vi "Duplicate_AO_WF.vi"(8 "error in (no error)":errorcluster) -> (0 "error out":errorcluster)   [LabVIEW 2025]
uses:
  <vilib>/Waveform/WDTOps.llb/WDT Append Waveforms DBL.vi
panel:
  out "AO WF":waveform(dbl)[](graph) caption="Output Waveform"
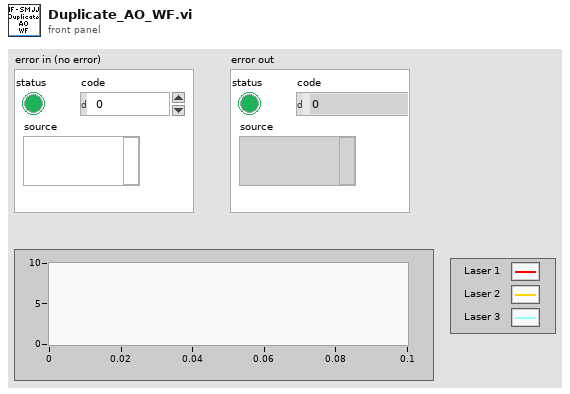
[diagram p1: front panel]
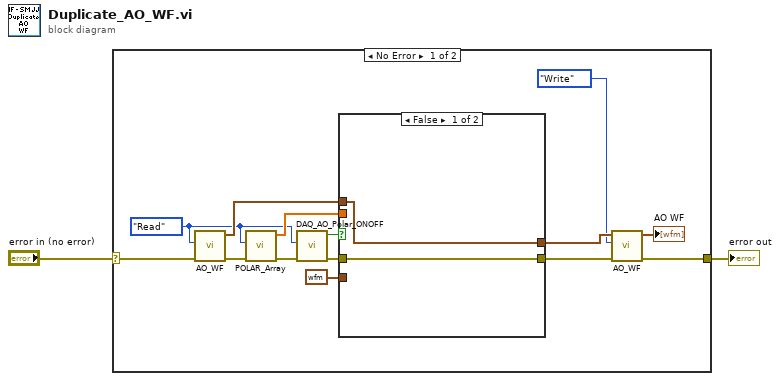
[diagram p0: block diagram]
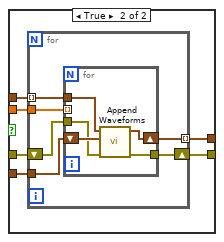
[diagram p2: hidden frame]
diagram:
  n1 = case shown="No Error" "error in (no error)" {
    selector: "error in (no error)" -> [w13 w36]
    tunnel: [w9 w36] -> w2
    frame No Error {
      w4 = enum16{"Init", "Write", "Read"}."Read" ("Action")
      n2 = call "AO_WF.vi"("error in"=w13, "Action"=w4) -> ("error out"=w14:errorcluster, "AO WF"=w15:waveform(dbl)[])  [unwired: 8 in]
      n3 = call "POLAR_Array.vi"("error in"=w14, "Action"=w4) -> ("error out"=w6:errorcluster, "Pockels_Array"=w16:dbl[])  [unwired: 8 in]
      n4 = call "DAQ_AO_Polar_ONOFF.vi"("error in"=w6, "Action"=w4) -> ("error out"=w5:errorcluster, "ON / OFF"=w3:bool)  [unwired: 8 in]
      n5 = case shown="False" w3 {
        tunnel: w16 -> [_ w24]
        tunnel: w15 -> [w18 w23]
        tunnel: [w18 w22] -> w12
        tunnel: [w17 w21] -> w10
        tunnel: waveform(i32) {"t0"=timestamp(0 s since 1904-01-01), "dt"=1.0, "Y"=[]} ("waveform out") -> [_ w20]
        tunnel: w5 -> [w17 w19]
        frame False {
        }
        frame True {
          n6 = for {
            tunnel: w24 -> [w29]
            tunnel: w23 -> [w28] mode=indexing
            tunnel: [w27] -> w22 mode=indexing
            tunnel: w20 -> [w25]
            shift-right: [w26] -> w21
            shift-left: w19 -> [w30]
            n7 = for {
              tunnel: w28 -> [w33]
              shift-right: [w35] -> w27
              shift-left: w25 -> [w34]
              tunnel: w30 -> [w32]
              tunnel: [w31] -> w26
              tunnel: w29 -> [_] mode=indexing
              n8 = call-poly <vilib>:"Append Waveforms.vi"("error in (no error)"=w32, "waveform B"=w34, "waveform A"=w33) -> ("error out"=w31:errorcluster, "waveform out"=w35:waveform(dbl))  [unwired: 7 in]
            }
          }
        }
      }
      n9 = call "AO_WF.vi"("error in"=w10, "Action"=enum16{"Init", "Write", "Read"}."Write", "AO WF"=w12) -> ("error out"=w9:errorcluster, "AO WF"=→"AO WF":waveform(dbl)[])  [unwired: 7 in]
    }
    frame Error {
    }
  }
  "error out" <- w2
